vi "StartTask.vi"(8 "error in (no error)":errorcluster, 10 "Stop?":bool, 11 "DaqMx_Single in":refnum<class "DaqMx_Single.lvclass">) -> (0 "error out":errorcluster, 3 "DaqMx_Single out":refnum<class "DaqMx_Single.lvclass">)   [LabVIEW 2014, in "FgenPlugins.lvlib" / "DaqMx_Single.lvclass"]
uses:
  DaqMx_Single.lvclass
  DaqMx_Single.lvclass/DaqMx_Single.ctl
  FgenPluginBaseClass/FgenPluginsBase.lvclass/FgenPluginsBase.ctl
  MemberClasses/FunctionBaseClass/FunctionBase.lvclass/FunctionBase.ctl
  Accessors/Write Running.vi
  FgenPluginBaseClass/Accessors/Read FunctionClass.vi
  MemberClasses/FunctionBaseClass/Accessors/Read Waveforms.vi
  MemberClasses/FunctionBaseClass/Accessors/Write Waveforms.vi
  FgenPluginBaseClass/Accessors/Write FunctionClass.vi
  Accessors/Read Running.vi
  MemberClasses/FunctionBaseClass/FunctionBase.lvclass
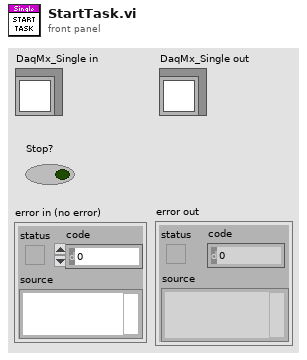
[diagram p1: front panel]
types:
  T1 = typedef "FgenPlugins.lvlib/Channel.ctl" = cluster{"Name":string, "Enabled":bool, "Operation":enum16{"Continuous", "Burst"}, "Impedance (50)":dbl, "Handle":string, "Connected":bool, "Mode (Function)":enum16{"Function", "Arbitrary", "Sequence"}}
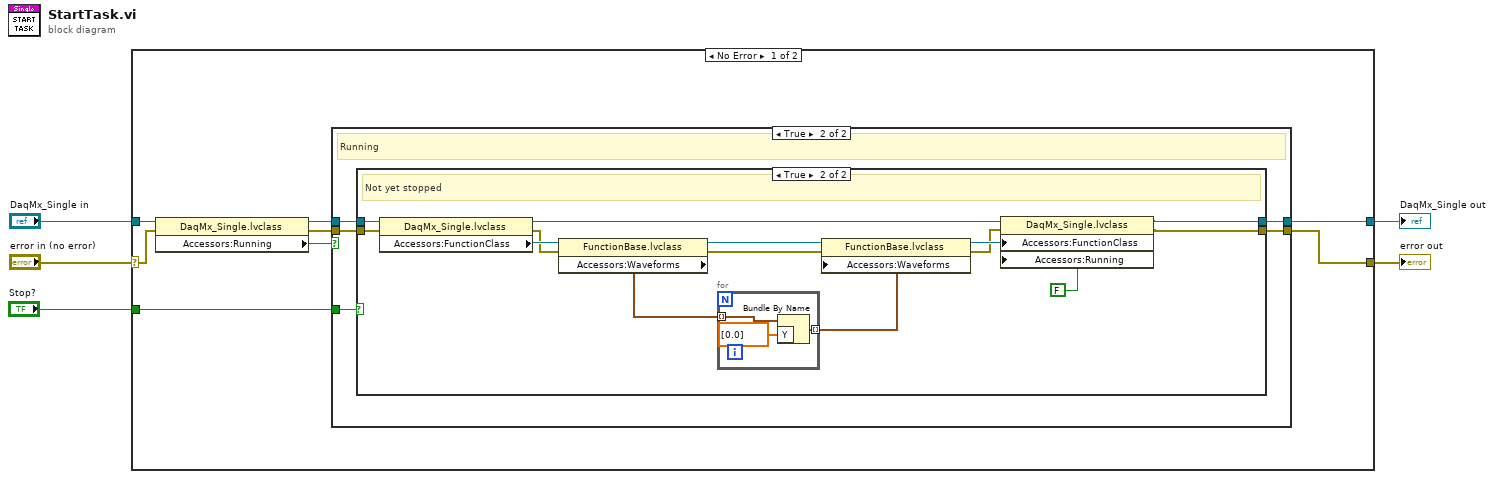
[diagram p0: block diagram]
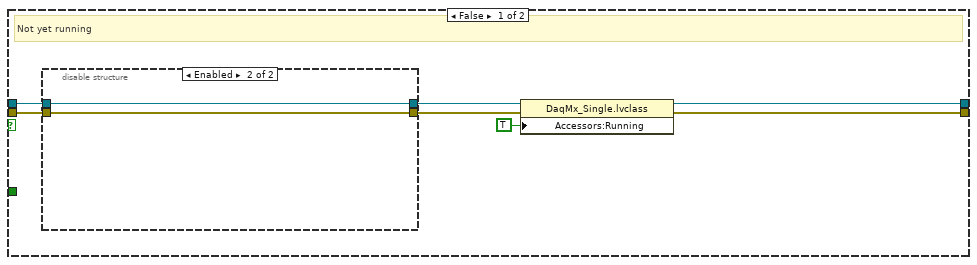
[diagram p2: hidden frame]
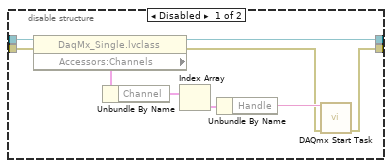
[diagram p3: hidden frame]
diagram:
  n1 = case shown="No Error" "error in (no error)" {
    selector: "error in (no error)" -> [w8 w57]
    tunnel: [w6 w57] -> w4
    tunnel: [w9 w56] -> w2
    tunnel: "DaqMx_Single in" -> [w13 w56]
    tunnel: "Stop?" -> [w11 _]
    frame No Error {
      n2 = property class="DaqMx_Single.lvclass"(reference=w13, error in=w8) -> (reference out=w10:refnum<class "DaqMx_Single.lvclass">, error out=w7:errorcluster, "Accessors:Running"=w12:bool)
      n3 = case shown="True" w12 {
        tunnel: w11 -> [_ w36]
        tunnel: w7 -> [w16 w33]
        tunnel: w10 -> [w17 w35]
        tunnel: [w20 w34] -> w9
        tunnel: [w18 w32] -> w6
        frame False {
          # "Not yet running"
          n4 = disable-structure shown="Enabled" {
            disable-tunnel: w17 -> [w27 w31]
            disable-tunnel: w16 -> [w26 w30]
            disable-tunnel: [w22 w30] -> w15
            disable-tunnel: [w21 w31] -> w14
            frame Disabled {
              n5 = property class="DaqMx_Single.lvclass"(reference=w27, error in=w26) -> (reference out=w21:refnum<class "DaqMx_Single.lvclass">, error out=w23:errorcluster, "Accessors:Channels"=w24:cluster{"Count":u16, "Channel":T1[]})
              n6 = Unbundle By Name(w24) -> ("Channel"=w29:T1[])
              n7 = Index Array(array=w29) -> (element=w28:T1)  [unwired: 1 in]
              n8 = Unbundle By Name(w28) -> ("Handle"=w25:string)
              n9 = call <vilib>:"DAQmx Start Task.vi"("task/channels in"=w25, "error in"=w23) -> ("error out"=w22:errorcluster)  [unwired: 12 in, 1 out]
            }
            frame Enabled {
            }
          }
          n10 = property class="DaqMx_Single.lvclass"(reference=w14, error in=w15, "Accessors:Running"=TRUE ("Running")) -> (reference out=w20:refnum<class "DaqMx_Single.lvclass">, error out=w18:errorcluster)
        }
        frame True {
          # "Running"
          n11 = case shown="True" w36 {
            tunnel: w35 -> [w37 w52]
            tunnel: [w37 w44] -> w34
            tunnel: w33 -> [w38 w51]
            tunnel: [w38 w43] -> w32
            frame False {
              # "Don't stop"
            }
            frame True {
              # "Not yet stopped"
              n12 = property class="DaqMx_Single.lvclass"(reference=w52, error in=w51) -> (reference out=w50:refnum<class "DaqMx_Single.lvclass">, error out=w46:errorcluster, "Accessors:FunctionClass"=w48:refnum<class "FunctionBase.lvclass">)
              n13 = property class="FunctionBase.lvclass"(reference=w48, error in=w46) -> (reference out=w42:refnum<class "FunctionBase.lvclass">, error out=w41:errorcluster, "Accessors:Waveforms"=w47:waveform(dbl)[])
              n14 = for {
                tunnel: w47 -> [w55] mode=indexing
                tunnel: [w53] -> w45 mode=indexing
                n15 = Bundle By Name(cluster=w55, "Y"=dbl[] [0.0]) -> (w53:waveform(dbl))
              }
              n16 = property class="FunctionBase.lvclass"(reference=w42, error in=w41, "Accessors:Waveforms"=w45) -> (reference out=w40:refnum<class "FunctionBase.lvclass">, error out=w39:errorcluster)
              n17 = property class="DaqMx_Single.lvclass"(reference=w50, error in=w39, "Accessors:FunctionClass"=w40, "Accessors:Running"=FALSE ("Running")) -> (reference out=w44:refnum<class "DaqMx_Single.lvclass">, error out=w43:errorcluster)
            }
          }
        }
      }
    }
    frame Error {
    }
  }
  "error out" <- w4
  "DaqMx_Single out" <- w2
